vi "Buffer Data.vi"(8 "error in (no error)":errorcluster, 9 "Time Stamp (Now)":timestamp, 10 "Data":dbl[](array[numeric]), 11 "Data Buffer in":refnum<class "Data Buffer DBL.lvclass">) -> (0 "error out":errorcluster, 3 "Data Buffer out":refnum<class "Data Buffer DBL.lvclass">)   [LabVIEW 2020, in "VolatusData.lvlib" / "Data Buffer DBL.lvclass"]
uses:
  Data Buffer DBL.lvclass
  Data Buffer DBL.lvclass/Data Buffer DBL.ctl
  VolatusData.lvlib
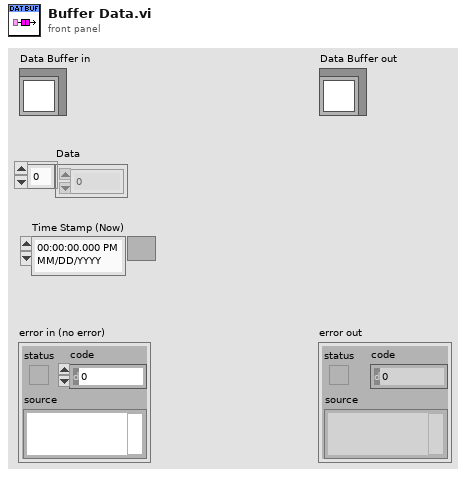
[diagram p1: front panel]
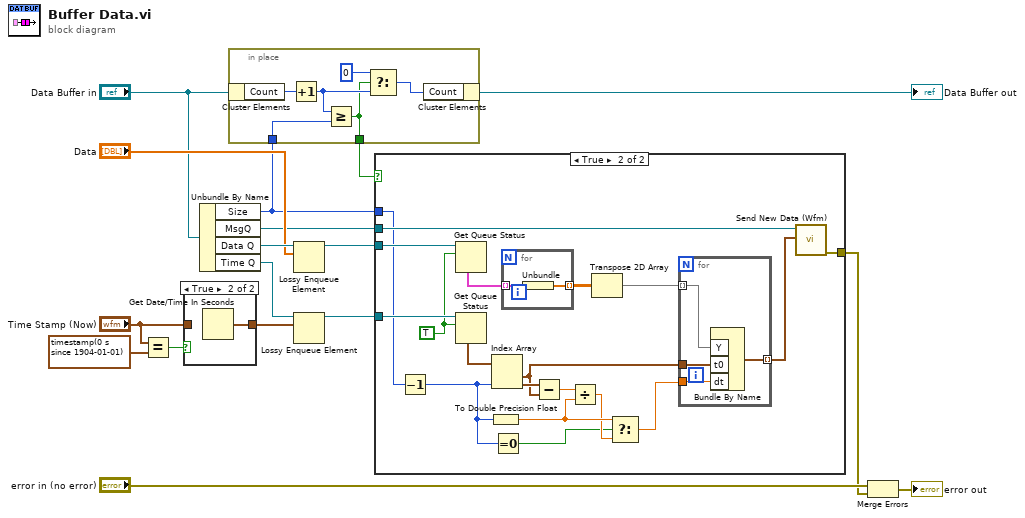
[diagram p0: block diagram]
diagram:
  n1 = Equal?(x="Time Stamp (Now)", y=timestamp(0 s since 1904-01-01)) -> (x = y?=w3:bool)
  n2 = case shown="True" w3 {
    tunnel: [w18 w19] -> w2
    tunnel: "Time Stamp (Now)" -> [w18 _]
    frame False {
    }
    frame True {
      n3 = Get Date/Time In Seconds() -> (seconds since 1Jan1904=w19:timestamp)
    }
  }
  n4 = Unbundle By Name("Data Buffer in") -> ("Size"=w5:i32, "MsgQ"=w10:refnum<class "MessageQ.lvclass">, "Data Q"=w16:refnum<queue>, "Time Q"=w15:refnum<queue>)
  n5 = in-place {
    in-place-border: w5 -> [w24]
    in-place-border: [w22] -> w11
    n6 = in-place-cluster #1("Data Buffer in") -> ("Count"=w25:i32)
    n7 = Increment(x=w25) -> (x+1=w23:i32)
    n8 = Greater Or Equal?(x=w23, y=w24) -> (x >= y?=w22:bool)
    n9 = Select(t=0, s=w22, f=w23) -> (s? t:f=w20:i32)
    n10 = in-place-cluster #1("Count"=w20) -> (→"Data Buffer out":refnum<class "Data Buffer DBL.lvclass">)
  }
  n11 = Lossy Enqueue Element(queue=w16, element="Data") -> (queue out=w9:refnum<queue>)  [unwired: 1 in, 3 out]
  n12 = Lossy Enqueue Element(queue=w15, element=w2) -> (queue out=w8:refnum<queue>)  [unwired: 1 in, 3 out]
  n13 = case shown="True" w11 {
    tunnel: w10 -> [_ w42]
    tunnel: w9 -> [_ w44]
    tunnel: w8 -> [_ w43]
    tunnel: [_ w41] -> w6
    tunnel: w5 -> [_ w39]
    frame False {
    }
    frame True {
      w40 = TRUE ("return elements? (F)")
      n14 = Decrement(x=w39) -> (x-1=w30:i32)
      n15 = Get Queue Status(queue=w44, return elements? (F)=w40) -> (elements=w33:cluster{dbl[]}[])  [unwired: 1 in, 7 out]
      n16 = Get Queue Status(queue=w43, return elements? (F)=w40) -> (elements=w37:timestamp[])  [unwired: 1 in, 7 out]
      n17 = To Double Precision Float(number=w30) -> (double precision float=w29:dbl)
      n18 = Index Array(array=w37, index #2=w30) -> (element #1=w35:timestamp, element #2=w36:timestamp)  [unwired: 1 in]
      n19 = Equal To 0?(x=w30) -> (x = 0?=w27:bool)
      n20 = for {
        tunnel: w33 -> [w46] mode=indexing
        tunnel: [w45] -> w32 mode=indexing
        n21 = Unbundle(w46) -> (w45:dbl[])
      }
      n22 = Subtract(x=w36, y=w35) -> (x-y=w38:dbl)
      n23 = Divide(x=w38, y=w29) -> (x/y=w28:dbl)
      n24 = Transpose 2D Array(2D array=w32) -> (transposed array=w31:dbl[][])
      n25 = Select(t=w29, s=w27, f=w28) -> (s? t:f=w26:dbl)
      n26 = for {
        tunnel: w26 -> [w49]
        tunnel: w35 -> [w50]
        tunnel: [w48] -> w34 mode=indexing
        tunnel: w31 -> [w47] mode=indexing
        n27 = Bundle By Name("Y"=w47, "t0"=w50, "dt"=w49) -> (w48:waveform(dbl))  [unwired: 1 in]
      }
      n28 = call "Send New Data (Wfm).vi"("Channels"=w34, "MessageQ"=w42) -> ("error out"=w41:errorcluster)  [unwired: 9 in]
    }
  }
  n29 = Merge Errors("error in (no error)", w6) -> (→"error out":errorcluster)
